vi "crio_9073_FPGA_Load_Cell.vi"() -> ()   [LabVIEW 2019]
uses:
  <vilib>/LabVIEW Targets/FPGA/cRIO/shared/nicrio_ModuleControls/nicrio_cRIO-9237_DataRatesRing.ctl
  <vilib>/LabVIEW Targets/FPGA/cRIO/shared/nicrio_ModuleControls/nicrio_cRIO-9237_ExcitationVoltageRing.ctl
  <vilib>/rvi/Emulation/niFpgaSctlEmulationGetInTimedLoop.vi
  <vilib>/rvi/Emulation/niFpgaProcessEmulError.vi
  <vilib>/rvi/eio/common/nirviEmuTemplatePropertySet_errors.vi
  <vilib>/rvi/eio/common/nirviEmuTemplateMethod_errors.vi
  <vilib>/rvi/Emulation/niFpgaGetClockAttributes.vi
  <vilib>/rvi/Emulation/niFpgaEmulationReportErrorSimple.vi
  <vilib>/rvi/Emulation/niFpgaCriticalErrorInLSC.vi
  <vilib>/eio/EIOPropertyNode/EIOPropertyNode.xnode
  <vilib>/eio/EIONode/EIONode.xnode
  <vilib>/rvi/eio/common/nirviEmuTemplatePropertyGet_errors.vi
  <vilib>/rvi/eio/common/nirviEmuTemplatePropertyGet_noerrors.vi
  <vilib>/rvi/eio/common/nirviEmuTemplatePropertySet_noerrors.vi
panel:
  out "Mod1/AI0":fxp<+/-,24,-4>
  in  "Half-Bridge Enable":bool
  in  "Excitation Voltage":T1 items=["2.5 Volts", "3.3 Volts", "5.0 Volts", "10.0 Volts", "External Excitation"]
  in  "Finite?":bool=TRUE
  in  "Samples per Channel":u32=1000
  in  "Shunt Cal Enable":bool
  in  "Stop Button":bool
  in  "Data Rate":T2=1 items=["50.000 kS/s (NI 9237)"=1, "25.000 kS/s (NI 9237)"=2, "16.667 kS/s (NI 9237)"=3, "12.500 kS/s (NI 9237)"=4, "10.000 kS/s (NI 9237)"=5, "8.333 kS/s (NI 9237)"=6, "7.143 kS/s (NI 9237)"=7, "6.250 kS/s (NI 9237)"=8, "5.556 kS/s (NI 9237)"=9, "5.000 kS/s (NI 9237)"=10, "4.545 kS/s (NI 9237)"=11, "4.167 kS/s (NI 9237)"=12, "3.846 kS/s (NI 9237)"=13, "3.571 kS/s (NI 9237)"=14, "3.333 kS/s (NI 9237)"=15, "3.125 kS/s (NI 9237)"=16, "2.941 kS/s (NI 9237)"=17, "2.778 kS/s (NI 9237)"=18, "2.632 kS/s (NI 9237)"=19, "2.500 kS/s (NI 9237)"=20, "2.381 kS/s (NI 9237)"=21, "2.273 kS/s (NI 9237)"=22, "2.174 kS/s (NI 9237)"=23, "2.083 kS/s (NI 9237)"=24, "2.000 kS/s (NI 9237)"=25, "1.923 kS/s (NI 9237)"=26, "1.852 kS/s (NI 9237)"=27, "1.786 kS/s (NI 9237)"=28, "1.724 kS/s (NI 9237)"=29, "1.667 kS/s (NI 9237)"=30, "1.613 kS/s (NI 9237)"=31]
  out "error out":errorcluster {"code" format="%.0x"}
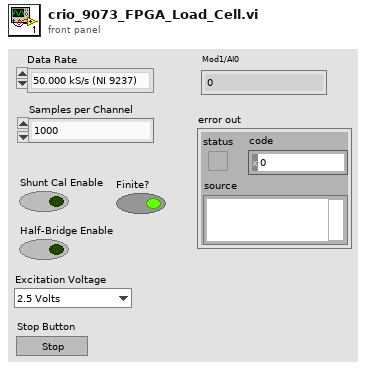
[diagram p1: front panel]
types:
  T1 = typedef "nicrio_cRIO-9237_ExcitationVoltageRing.ctl" = u8
  T2 = typedef "nicrio_cRIO-9237_DataRatesRing.ctl" = u8
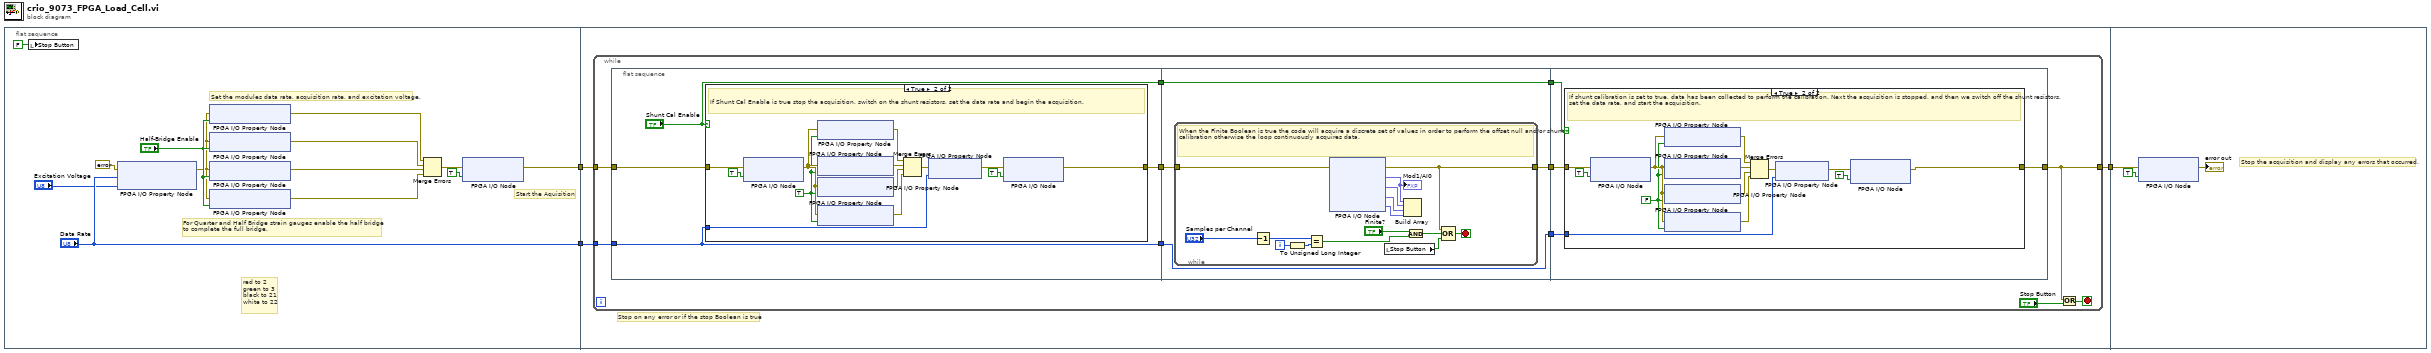
[diagram p0: block diagram]
diagram:
  n1 = flat-sequence {
    tunnel: [w15] -> w3
    tunnel: ["Data Rate"] -> w2
    tunnel: w3 -> [w19]
    tunnel: w2 -> [w18]
    tunnel: [w17] -> w1
    tunnel: w1 -> [w87]
    frame #0 {
      # "red to 2\ngreen to 3\nblack to 21\nwhite to 22"
      # "Start the Aquisition"
      # "For Quarter and Half Bridge strain gauges enable the half bridge \nto complete the full bridge."
      # "Set the modules data rate, acquisition rate, and excitation voltage."
      n2 = local write "Stop Button"(FALSE ("Stop Button")) -> ()
      n3 = xnode "FPGA I/O Property Node"("error in"=errorcluster {"status"=FALSE, "code"=0, "source"=""}, "Data Rate"="Data Rate", "Excitation Voltage"="Excitation Voltage") -> ("error out"=w6:errorcluster)  [unwired: 1 in, 1 out]
      n4 = xnode "FPGA I/O Property Node"("error in"=w6, "Half-Bridge Enable"="Half-Bridge Enable") -> ("error out"=w10:errorcluster)  [unwired: 1 in, 1 out]
      n5 = xnode "FPGA I/O Property Node"("error in"=w6, "Half-Bridge Enable"="Half-Bridge Enable") -> ("error out"=w9:errorcluster)  [unwired: 1 in, 1 out]
      n6 = xnode "FPGA I/O Property Node"("error in"=w6, "Half-Bridge Enable"="Half-Bridge Enable") -> ("error out"=w8:errorcluster)  [unwired: 1 in, 1 out]
      n7 = xnode "FPGA I/O Property Node"("error in"=w6, "Half-Bridge Enable"="Half-Bridge Enable") -> ("error out"=w7:errorcluster)  [unwired: 1 in, 1 out]
      n8 = Merge Errors(w10, w9, w8, w7) -> (w5:errorcluster)
      n9 = xnode "FPGA I/O Node"("error in"=w5, "Mod1/Start"=TRUE ("Mod1/Stop")) -> ("error out"=w15:errorcluster)  [unwired: 1 in, 1 out]
    }
    frame #1 {
      # "Stop on any error or if the stop Boolean is true"
      n10 = while {
        tunnel: w19 -> [w30]
        tunnel: [w27] -> w17
        tunnel: w18 -> [w24]
        stop <- w28 stop-if-true
        n11 = flat-sequence {
          tunnel: [w33] -> w25
          tunnel: [w32] -> w22
          tunnel: ["Shunt Cal Enable"] -> w21
          tunnel: w24 -> [w32]
          tunnel: w30 -> [w34]
          tunnel: [w51] -> w29
          tunnel: w25 -> [w52]
          tunnel: [w50] -> w23
          tunnel: w22 -> [w50]
          tunnel: w21 -> [w49]
          tunnel: [w49] -> w20
          tunnel: [w70] -> w27
          tunnel: w29 -> [w71]
          tunnel: w23 -> [w68]
          tunnel: w20 -> [w69]
          frame #0 {
            n12 = case shown="True" "Shunt Cal Enable" {
              tunnel: w34 -> [w35 w45]
              tunnel: [w35 w43] -> w33
              tunnel: w32 -> [_ w40]
              frame False {
              }
              frame True {
                w38 = TRUE ("Shunt Cal Enable")
                # "If Shunt Cal Enable is true stop the acquisition, switch on the shunt resistors, set the data rate and begin the acquisition."
                n13 = xnode "FPGA I/O Node"("error in"=w45, "Mod1/Stop"=TRUE) -> ("error out"=w44:errorcluster)  [unwired: 1 in, 1 out]
                n14 = xnode "FPGA I/O Property Node"("error in"=w44, "Shunt Cal Enable"=w38) -> ("error out"=w48:errorcluster)  [unwired: 1 in, 1 out]
                n15 = xnode "FPGA I/O Property Node"("error in"=w44, "Shunt Cal Enable"=w38) -> ("error out"=w36:errorcluster)  [unwired: 1 in, 1 out]
                n16 = xnode "FPGA I/O Property Node"("error in"=w44, "Shunt Cal Enable"=w38) -> ("error out"=w47:errorcluster)  [unwired: 1 in, 1 out]
                n17 = xnode "FPGA I/O Property Node"("error in"=w44, "Shunt Cal Enable"=w38) -> ("error out"=w46:errorcluster)  [unwired: 1 in, 1 out]
                n18 = Merge Errors(w48, w36, w47, w46) -> (w41:errorcluster)
                n19 = xnode "FPGA I/O Property Node"("error in"=w41, "Data Rate"=w40) -> ("error out"=w42:errorcluster)  [unwired: 1 in, 1 out]
                n20 = xnode "FPGA I/O Node"("error in"=w42, "Mod1/Start"=TRUE) -> ("error out"=w43:errorcluster)  [unwired: 1 in, 1 out]
              }
            }
          }
          frame #1 {
            n21 = while {
              tunnel: w52 -> [w53]
              tunnel: [w57] -> w51
              i -> [w61]
              stop <- w54 stop-if-true
              # "When the Finite Boolean is true the code will acquire a discrete set of values in order to perform the offset null and/or shunt calibration otherwise the loop continuously acquires data."
              n22 = Decrement(x="Samples per Channel") -> (x-1=w63:u32)
              n23 = To Unsigned Long Integer(number=w61) -> (unsigned 32bit integer=w62:u32)
              n24 = Equal?(x=w63, y=w62) -> (x = y?=w58:bool)
              n25 = xnode "FPGA I/O Node"("error in"=w53) -> ("error out"=w57:errorcluster, "Mod1/AI0"=w67:fxp<+/-,24,-4>, "Mod1/AI1"=w66:fxp<+/-,24,-4>, "Mod1/AI2"=w64:fxp<+/-,24,-4>, "Mod1/AI3"=w65:fxp<+/-,24,-4>)  [unwired: 4 in, 4 out]
              "Mod1/AI0" <- w67
              n26 = local read "Stop Button"() -> (w55:bool)
              n27 = Build Array(w67, w66, w64, w65) -> ()  [unwired: 1 out]
              n28 = And(x="Finite?", y=w58) -> (x .and. y?=w56:bool)
              n29 = Compound Arithmetic op=OR(w57, w56, w55) -> (w54:bool)
            }
          }
          frame #2 {
            n30 = case shown="True" w69 {
              tunnel: w71 -> [w72 w81]
              tunnel: [w72 w79] -> w70
              tunnel: w68 -> [_ w76]
              frame False {
              }
              frame True {
                w75 = FALSE ("Shunt Cal Enable")
                # "If shunt calibration is set to true, data has been collected to perform the calibration. Next the acquisition is stopped, and then we switch off the shunt resistors, set the data rate, and start the acquisition."
                n31 = xnode "FPGA I/O Node"("error in"=w81, "Mod1/Stop"=TRUE) -> ("error out"=w80:errorcluster)  [unwired: 1 in, 1 out]
                n32 = xnode "FPGA I/O Property Node"("error in"=w80, "Shunt Cal Enable"=w75) -> ("error out"=w85:errorcluster)  [unwired: 1 in, 1 out]
                n33 = xnode "FPGA I/O Property Node"("error in"=w80, "Shunt Cal Enable"=w75) -> ("error out"=w84:errorcluster)  [unwired: 1 in, 1 out]
                n34 = xnode "FPGA I/O Property Node"("error in"=w80, "Shunt Cal Enable"=w75) -> ("error out"=w83:errorcluster)  [unwired: 1 in, 1 out]
                n35 = xnode "FPGA I/O Property Node"("error in"=w80, "Shunt Cal Enable"=w75) -> ("error out"=w82:errorcluster)  [unwired: 1 in, 1 out]
                n36 = Merge Errors(w85, w84, w83, w82) -> (w77:errorcluster)
                n37 = xnode "FPGA I/O Property Node"("error in"=w77, "Data Rate"=w76) -> ("error out"=w78:errorcluster)  [unwired: 1 in, 1 out]
                n38 = xnode "FPGA I/O Node"("error in"=w78, "Mod1/Start"=TRUE) -> ("error out"=w79:errorcluster)  [unwired: 1 in, 1 out]
              }
            }
          }
        }
        n39 = Or(x=w27, y="Stop Button") -> (x .or. y?=w28:bool)
      }
    }
    frame #2 {
      # "Stop the acquisition and display any errors that occurred."
      n40 = xnode "FPGA I/O Node"("error in"=w87, "Mod1/Stop"=TRUE) -> ("error out"=→"error out":errorcluster)  [unwired: 1 in, 1 out]
    }
  }
